vi "EXO_System.vi"() -> ()   [LabVIEW 2012]
uses:
  <vilib>/Platform/TimedLoop/XDataNode/timing_clust.ctl
  <vilib>/Platform/TimedLoop/XDataNode/nitl_modes.ctl
  <vilib>/Platform/TimedLoop/XDataNode/wakeup.ctl
  <vilib>/addons/database/Connection.llb/DB Tools Open Connec (Path).vi
  SubVi's/Connection Variable Common.vi
  SlowCtrl/LabView ESIII/LabView ESIII/Data grabber Folder/Documents and Settings/loaner/Desktop/Desktop/LabView Dec/LabView Dec.8/SubVi's/Plot Variable.vi
  SubVi's/Cryopump Variable.vi
  SubVi's/Monitor B Variable.vi
  SlowCtrl/LabView ESIII/LabView ESIII/SubVi's/Time Zone Offset.vi
  SlowCtrl/LabView ESIII/LabView ESIII/SubVi's/Time Variable.vi
  SlowCtrl/LabView ESIII/LabView ESIII/SubVi's/Connection Variable 1.vi
  <vilib>/Platform/TimedLoop/XDataNode/XDataNode.xnode
  <vilib>/Platform/TimedLoop/XDataNode/XDNodeRunTimeDep.lvlib
  <vilib>/addons/database/NI_Database_API.lvlib
panel:
  out "Version out of date?":bool
  out "ESIII":bool
  in  "Quit Button":bool
  in  "Plot and Fit":bool
  in  "EXO FrontPanel":bool
  # "ESIII EXO Gas Phase"
  # "Version: 2.26"
  # "Release Date: 9/3/10"
  # "Control/Monitoring Programs"
  # "Database:"
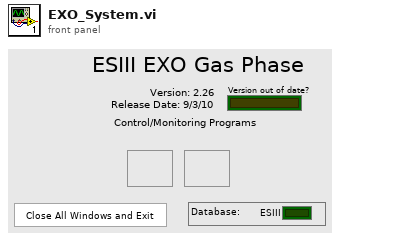
[diagram p1: front panel]
types:
  T1 = typedef "NI_Database_API.lvlib/Conn ObjectReference.ctl" = refnum<k1>
  T2 = typedef "XDNodeRunTimeDep.lvlib/timing_clust.ctl" = cluster{"Expected End [f-1]":u64, "Actual End [f-1]":u64, "Finished Late? [f-1]":bool, "Expected End [i-1]":u64, "Actual End [i-1]":u64, "Finished Late? [i-1]":bool, "Expected Start [i]":u64, "Actual Start [i]":u64, "Expected Start [f]":u64, "Actual Start [f]":u64, "Source Name":string, "Structure Name":string, "Period":i64, "Deadline":i64, "Offset":i64, "Start":i64, "Priority":i32, "Timeout":i32, "Mode":T3, "Wakeup Reason":T4, "Error":errorcluster, "Source Type":string, "Secondary Source Type":string, "Global End Time":u64, "Global Start Time":u64, "Frame Duration":u64, "Iteration Duration":u64, "Assigned CPU":i32, "I/O Scan Engine Mode":u32}
  T3 = typedef "XDNodeRunTimeDep.lvlib/nitl_modes.ctl" = enum32{"No Change", "Process missed periods, maintain original phase", "Discard missed periods, maintain original phase", "Process missed periods, ignore original phase", "Discard missed periods, ignore original phase"}
  T4 = typedef "XDNodeRunTimeDep.lvlib/wakeup.ctl" = enum32{"Normal", "Aborted", "Asynchronous wakeup", "Timing source error", "Timed loop error", "Timeout"}
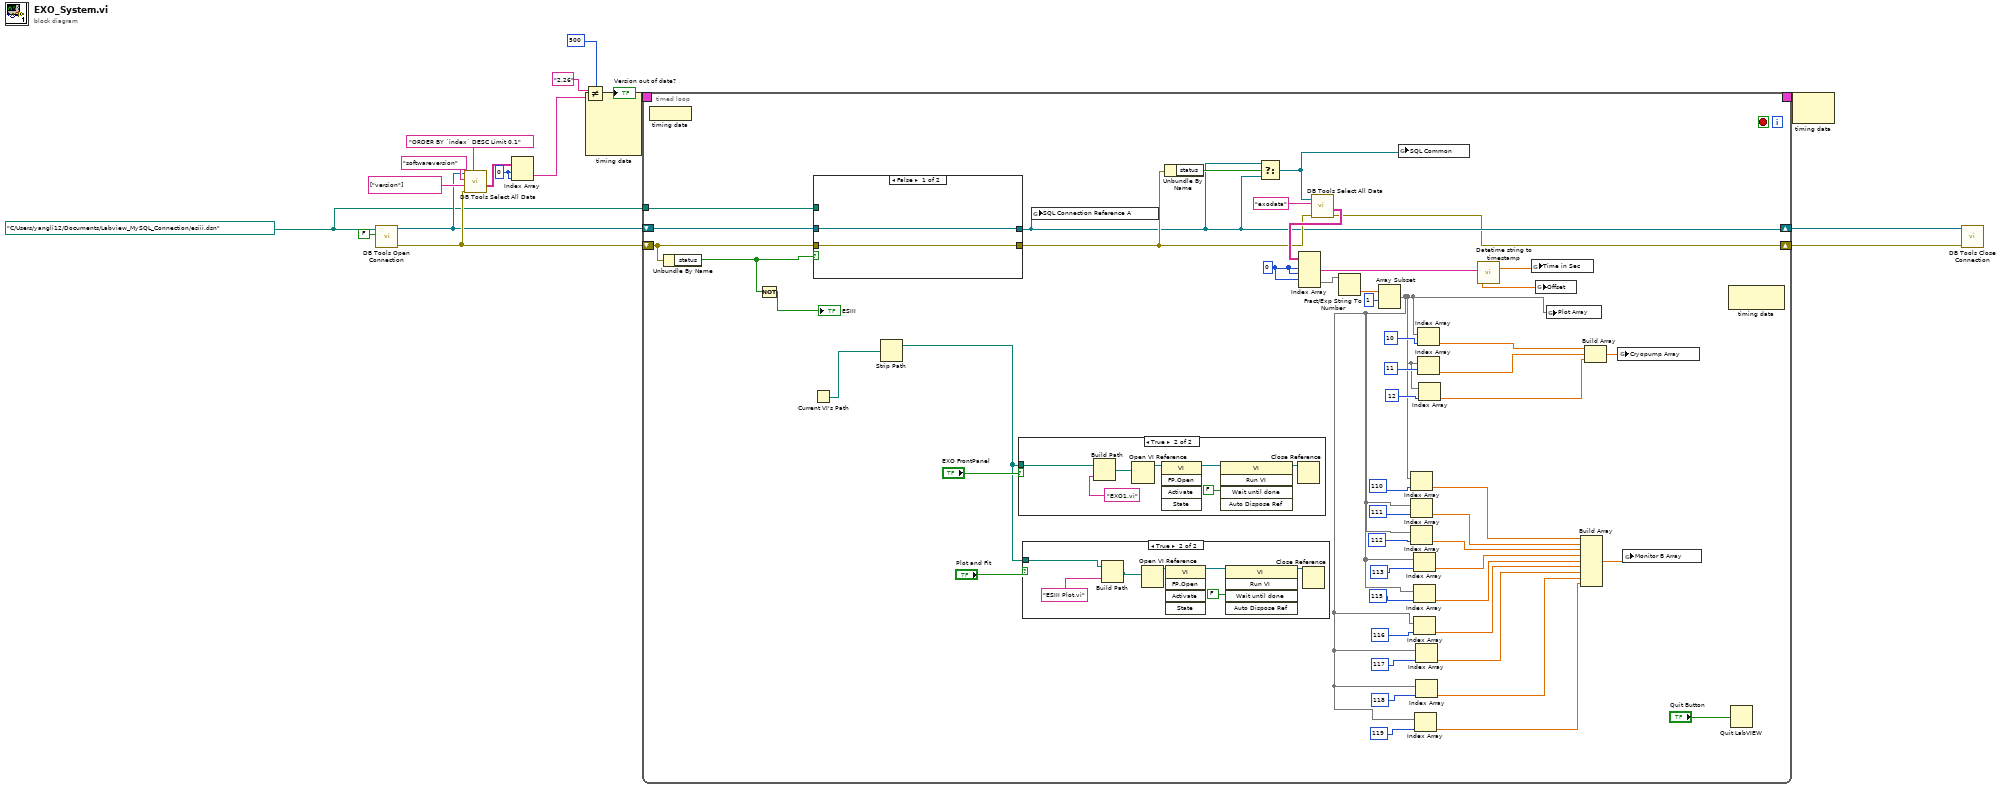
[diagram p0: block diagram]
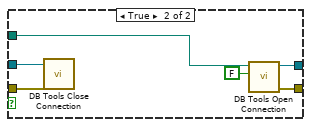
[diagram p2: hidden frame]
diagram:
  w2 = path "C:/Users/yangli12/Documents/Labview_MySQL_Connection/esiii.dsn" ("connection information")
  w4 = 0 ("index (row)")
  n1 = call-poly <vilib>:"DB Tools Open Connection.vi"("prompt? (F)"=FALSE, "connection information"=w2) -> ("error out"=w12:errorcluster, "connection reference"=w3:T1)  [unwired: 3 in, 3 out]
  n2 = call <vilib>:"DB Tools Select All Data.vi"("optional clause"="ORDER BY `index` DESC Limit 0,1", "error in (no error)"=w12, "columns"=string[] ["version"], "table"="softwareversion", "connection reference"=w3) -> ("data"=w8:string[][])  [unwired: 3 out]
  n3 = Index Array(array=w8, index (row)=w4, index (col)=w4) -> (element=w6:string)
  n4 = Not Equal?(x="2.26", y=w6) -> (x != y?=→"Version out of date?":bool)
  n5 = node-c288(i64 500 ("Period")) -> (w17:T2)  [unwired: 3 out]
  n6 = timed-loop {
    timing: w17 -> [_]
    timing-out: [_] -> w16
    shift-right: [w32] -> w14
    shift-left: w3 -> [w58]
    shift-right: [w26] -> w13
    shift-left: w12 -> [w50]
    tunnel: w2 -> [w51]
    stop <- _ stop-if-true
    w52 = 0 ("index (row)")
    n7 = node-c288 ("Output Node")() -> ()  [unwired: 1 out]
    n8 = Unbundle By Name(w50) -> ("status"=w37:bool)
    n9 = Not(x=w37) -> (.not. x?=→"ESIII":bool)
    n10 = Current VI's Path() -> (path=w60:path)
    n11 = case shown="False" w37 {
      tunnel: [w70 w76] -> w32
      tunnel: [w69 w75] -> w35
      tunnel: w58 -> [w70 w72]
      tunnel: w50 -> [w69 w73]
      tunnel: w51 -> [_ w74]
      frame False {
      }
      frame True {
        n12 = call <vilib>:"DB Tools Close Connection.vi"("error in (no error)"=w73, "connection reference"=w72) -> ()  [unwired: 6 out]
        n13 = call-poly <vilib>:"DB Tools Open Connection.vi"("prompt? (F)"=FALSE, "connection information"=w74) -> ("error out"=w75:errorcluster, "connection reference"=w76:T1)  [unwired: 3 in, 3 out]
      }
    }
    n14 = Strip Path(path=w60) -> (stripped path=w27:path)  [unwired: 1 out]
    n15 = case shown="True" "EXO FrontPanel" {
      tunnel: w27 -> [_ w86]
      frame False {
      }
      frame True {
        n16 = Build Path(base path=w86, name or relative path="EXO1.vi") -> (appended path=w84:path)
        n17 = Open VI Reference(vi path=w84) -> (vi reference=w90:refnum<vi>)  [unwired: 2 in, 4 out]
        n18 = invoke class="VI" method="FP.Open"(reference=w90) -> (reference out=w89:refnum<vi>)  [unwired: 4 in, 4 out]
        n19 = invoke class="VI" method="Run VI"(reference=w89, "Wait until done"=FALSE ("Wait Until Done")) -> (reference out=w88:refnum<vi>)  [unwired: 3 in, 4 out]
        n20 = Close Reference(reference=w88) -> ()  [unwired: 1 in, 1 out]
      }
    }
    n21 = case shown="True" "Plot and Fit" {
      tunnel: w27 -> [_ w77]
      frame False {
      }
      frame True {
        n22 = Build Path(base path=w77, name or relative path="ESIII Plot.vi") -> (appended path=w78:path)
        n23 = Open VI Reference(vi path=w78) -> (vi reference=w83:refnum<vi>)  [unwired: 1 in, 5 out]
        n24 = invoke class="VI" method="FP.Open"(reference=w83) -> (reference out=w82:refnum<vi>)  [unwired: 4 in, 4 out]
        n25 = invoke class="VI" method="Run VI"(reference=w82, "Wait until done"=FALSE ("Wait Until Done")) -> (reference out=w80:refnum<vi>)  [unwired: 3 in, 4 out]
        n26 = Close Reference(reference=w80) -> ()  [unwired: 1 in, 1 out]
      }
    }
    n27 = global write "Connection Variable 1.vi" "SQL Connection Reference A"(w32) -> ()
    n28 = Unbundle By Name(w35) -> ("status"=w46:bool)
    n29 = Select(t=w32, s=w46, f=w32) -> (s? t:f=w36:T1)
    n30 = call <vilib>:"DB Tools Select All Data.vi"("error in (no error)"=w35, "table"="exodata", "connection reference"=w36) -> ("error out"=w26:errorcluster, "data"=w56:string[][])  [unwired: 2 in, 2 out]
    n31 = Index Array(array=w56, index (row) #1=w52, index (col) #1=w52, index (row) #2=w52) -> (element #1=w39:string, element #2=w53:string[])  [unwired: 1 in]
    n32 = Fract/Exp String To Number(string=w53) -> (number=w55:dbl[])  [unwired: 4 out]
    n33 = Array Subset(array=w55, index=1) -> (w18:dbl[])  [unwired: 1 in]
    n34 = global write "Connection Variable Common.vi" "SQL Common"(w36) -> ()
    n35 = Index Array(array=w18, index=110) -> (element=w64:dbl)
    n36 = Index Array(array=w18, index=111) -> (element=w63:dbl)
    n37 = Index Array(array=w18, index=112) -> (element=w62:dbl)
    n38 = Index Array(array=w18, index=113) -> (element=w48:dbl)
    n39 = Index Array(array=w18, index=115 ("length")) -> (element=w44:dbl)
    n40 = Index Array(array=w18, index=116 ("length")) -> (element=w42:dbl)
    n41 = Index Array(array=w18, index=119) -> (element=w21:dbl)
    n42 = Index Array(array=w18, index=117) -> (element=w40:dbl)
    n43 = Index Array(array=w18, index=118) -> (element=w22:dbl)
    n44 = Index Array(array=w18, index=10 ("length")) -> (element=w29:dbl)
    n45 = Index Array(array=w18, index=11) -> (element=w34:dbl)
    n46 = Index Array(array=w18, index=12) -> (element=w19:dbl)
    n47 = call "Datetime string to timestamp.vi"("timestamp string"=w39) -> ("Time in sec"=w38:dbl, "Offset"=w25:dbl)  [unwired: 1 out]
    n48 = global write "Time Variable.vi" "Time in Sec"(w38) -> ()
    n49 = global write "Time Zone Offset.vi" "Offset"(w25) -> ()
    n50 = global write "Plot Variable.vi" "Plot Array"(w18) -> ()
    n51 = Build Array(w64, w63, w62, w48, w44, w42, w40, w22, w21) -> (w30:dbl[])
    n52 = Build Array(w29, w34, w19) -> (w31:dbl[])
    n53 = global write "Cryopump Variable.vi" "Cryopump Array"(w31) -> ()
    n54 = global write "Monitor B Variable.vi" "Monitor B Array"(w30) -> ()
    n55 = node-c288() -> ()  [unwired: 2 out]
    n56 = Quit LabVIEW(quit? (T)="Quit Button") -> ()
  }
  n57 = node-c288(w16) -> ()  [unwired: 1 out]
  n58 = call <vilib>:"DB Tools Close Connection.vi"("error in (no error)"=w13, "connection reference"=w14) -> ()  [unwired: 6 out]
